vi "ReadMicronConfig.vi"(8 "Error In":errorcluster, 10 "Mode":string, 11 "Micron Path In":path) -> (0 "Error Out":errorcluster, 3 "Micron Mode":T1)   [LabVIEW 2019, in "MicronClient.lvclass"]
uses:
  MicronClient.lvclass
  Typedefs/MicronModeINISection.ctl
  Typedefs/MicronINISection.ctl
  <vilib>/Utility/config.llb/NI_LVConfig.lvlib
  <vilib>/SLL Toolkit/SLL File IO/SLL File IO.lvlib
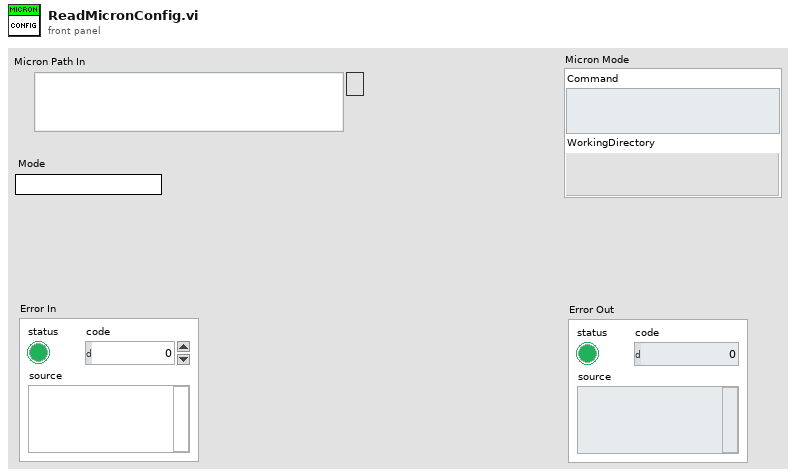
[diagram p1: front panel]
types:
  T1 = typedef "MicronClient.lvclass/MicronModeINISection.ctl" = cluster{"Command":string, "WorkingDirectory":path}
  T2 = typedef "MicronClient.lvclass/MicronINISection.ctl" = cluster{"Mode":string}
  T3 = typedef "NI_LVConfig.lvlib/Config Data RefNum.ctl" = refnum<k1>
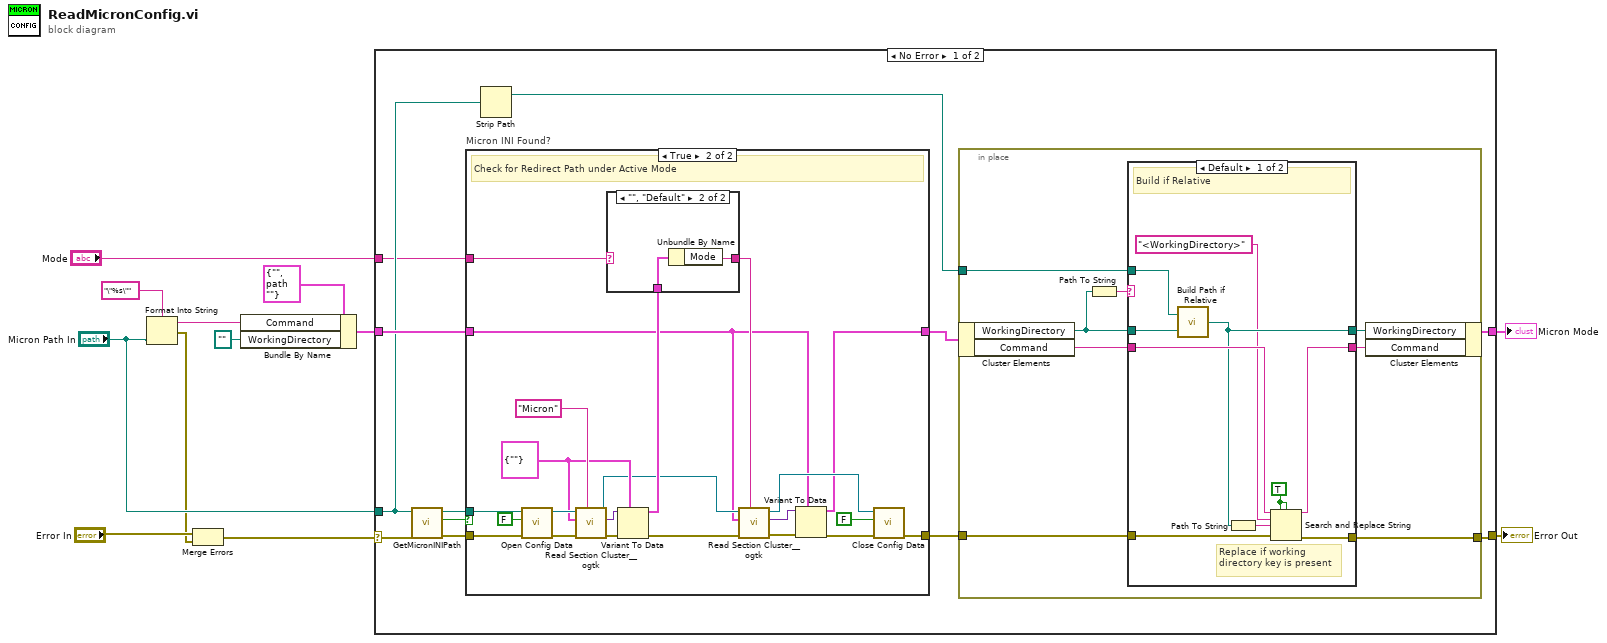
[diagram p0: block diagram]
diagram:
  n1 = Format Into String(format string="\"%s\"", "Micron Path In") -> (resulting string=w10:string, error out=w4:errorcluster)  [unwired: 2 in]
  n2 = Merge Errors("Error In", w4) -> (w3:errorcluster)
  n3 = Bundle By Name(cluster=T1 {"Command"="", "WorkingDirectory"=path ""} ("Micron Mode"), "Command"=w10, "WorkingDirectory"=path "") -> (w6:T1)
  n4 = case shown="No Error" w3 {
    selector: w3 -> [w20 w74]
    tunnel: "Micron Path In" -> [w17 _]
    tunnel: [w13 w74] -> w11
    tunnel: w6 -> [w21 w73]
    tunnel: [w18 w73] -> w2
    tunnel: "Mode" -> [w15 _]
    frame No Error {
      n5 = call "GetMicronINIPath.vi"("Error In"=w20, "Micron Path In"=w17) -> ("Error Out"=w24:errorcluster, "Present?"=w22:bool, "Micron INI Path Out"=w23:path)  [unwired: 7 in]
      n6 = case "Micron INI Found?" shown="True" w22 {
        tunnel: w24 -> [w47 w69]
        tunnel: w23 -> [_ w51]
        tunnel: [w47 w52] -> w14
        tunnel: [w46 w50] -> w19
        tunnel: w21 -> [w46 w49]
        tunnel: w15 -> [_ w48]
        frame False {
        }
        frame True {
          w62 = T2 {"Mode"=""} ("Micron")
          # "Check for Redirect Path under Active Mode"
          n7 = call <vilib>:"Open Config Data.vi"("error in (no error)"=w69, "create file if necessary (T)"=FALSE, "configuration file path"=w51) -> ("error out"=w68:errorcluster, "refnum"=w65:T3)  [unwired: 6 in, 1 out]
          n8 = call <userlib>:"Read Section Cluster__ogtk.vi"("section (optional)"="Micron", "error in (no error)"=w68, "Section Formatted Cluster Type"=w62, "refnum"=w65) -> ("error out"=w66:errorcluster, "Section Formatted Cluster"=w63:variant, "dup refnum"=w59:T3)  [unwired: 3 in, 2 out]
          n9 = Variant To Data(error in=w66, type=w62, Variant=w63) -> (data=w61:T2, error out=w60:errorcluster)
          n10 = case shown="\"\", \"Default\"" w48 {
            selector: w48 -> [w70 _]
            tunnel: w61 -> [_ w72]
            tunnel: [w70 w71] -> w58
            frame Default {
              # "Mode over-ridden by passed in value"
            }
            frame "", "Default" {
              n11 = Unbundle By Name(w72) -> ("Mode"=w71:string)
            }
          }
          n12 = call <userlib>:"Read Section Cluster__ogtk.vi"("section (optional)"=w58, "error in (no error)"=w60, "Section Formatted Cluster Type"=w49, "refnum"=w59) -> ("error out"=w57:errorcluster, "Section Formatted Cluster"=w56:variant, "dup refnum"=w54:T3)  [unwired: 3 in, 2 out]
          n13 = Variant To Data(error in=w57, type=w49, Variant=w56) -> (data=w50:T1, error out=w55:errorcluster)
          n14 = call <vilib>:"Close Config Data.vi"("error in (no error)"=w55, "write file if changed (T)"=FALSE, "refnum"=w54) -> ("error out"=w52:errorcluster)  [unwired: 7 in, 1 out]
        }
      }
      n15 = Strip Path(path=w17) -> (stripped path=w16:path)  [unwired: 1 out]
      n16 = in-place {
        in-place-border: w16 -> [w29]
        in-place-border: w14 -> [w26]
        in-place-border: [w25] -> w13
        n17 = in-place-cluster #1(w19) -> ("WorkingDirectory"=w31:path, "Command"=w28:string)
        n18 = Path To String(path=w31) -> (string=w32:string)
        n19 = case shown="Default" w32 {
          tunnel: w31 -> [w42 w45]
          tunnel: [w35 w45] -> w30
          tunnel: w29 -> [w41 _]
          tunnel: w28 -> [w40 w43]
          tunnel: [w39 w43] -> w27
          tunnel: w26 -> [w37 w44]
          tunnel: [w36 w44] -> w25
          frame Default {
            w38 = TRUE ("replace all? (F)")
            # "Replace if working directory key is present"
            # "Build if Relative"
            n20 = call <vilib>:"Build Path if Relative.vi"("Relative or Absolute Path"=w42, "Base Path"=w41) -> ("Path Out"=w35:path)
            n21 = Path To String(path=w35) -> (string=w34:string)
            n22 = Search and Replace String(replace all?=w38, case sensitive?=w38, input string=w40, search string="<WorkingDirectory>", replace string=w34, error in=w37) -> (result string=w39:string, error out=w36:errorcluster)  [unwired: 2 in, 2 out]
          }
          frame "." {
          }
        }
        n23 = in-place-cluster #1("WorkingDirectory"=w30, "Command"=w27) -> (w18:T1)
      }
    }
    frame Error {
    }
  }
  "Error Out" <- w11
  "Micron Mode" <- w2
